vi "getLecServerList.vi"(8 "error in (no error)":errorcluster, 11 "SM1000-control in":T2) -> (0 "error out":errorcluster, 1 "Device identifiers":T1[](array[typedef]), 2 "piServerCount":i32, 3 "SM1000-control out":T2)   [LabVIEW 2013, in "SLMControl.lvlib" / "SM1000.lvclass"]
doc: "Get embedded controller device data.\n\nThis method returns a list of identifiers for the EC1000 modules for which valid broadcast packets have been received. One of the friendly names can be used in the method 'getBroadcastData' to obtain more extensive identification data.\nBecause of the asynchronous and periodic nature of the broadcast transmissions, it may take some time before all EC1000 controllers are recognized and reported via this method. Several successive calls may yield different results until enough time has passed to account for the longest broadcast interval. The broadcast interval is configured using the 'Session.requestFixedData' and 'Session.setFixedData' methods with the 'AdminConfig' data as an argument."
uses:
  SM1000.lvclass
  Object-reference.ctl
  Device-identification.ctl
  SM1000.lvclass/SM1000.ctl
  Custom-errors.ctl
  C:/Users/vangeste/Desktop/2015-06-02 - SLM - MAIF/HC-HardwareCharacterization/Sources/SM1000/LECBroadcast.dll
  HC-HardwareCharacterization/Sources/SM1000/LECBroadcast.dll
  DOTNET-error-int.vi
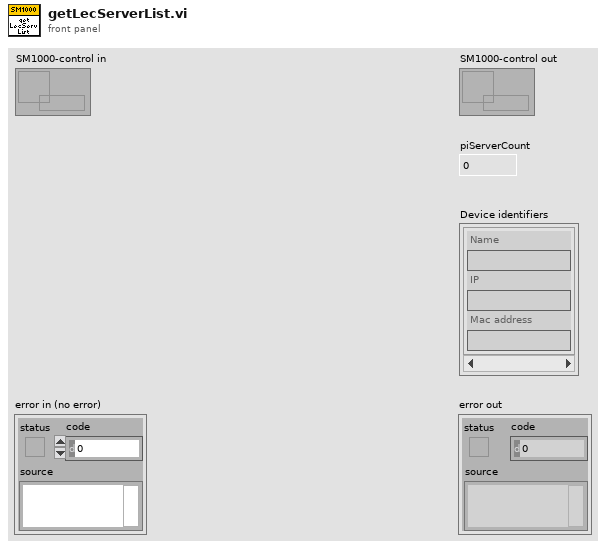
[diagram p1: front panel]
types:
  T1 = typedef "SLMControl.lvlib/SM1000.lvclass/Device-identification.ctl" = cluster{"Name":string, "IP":string, "Mac address":string}
  T2 = typedef "SLMControl.lvlib/SM1000.lvclass/Object-reference.ctl" = refnum<data-value>
  T3 = typedef "SLMControl.lvlib/SM1000.lvclass/Custom-errors.ctl" = enum16{"No error", "Not implemented", "Command not recognized", "Invalid input", "No connection", "Timeout", "Resource not loaded"}
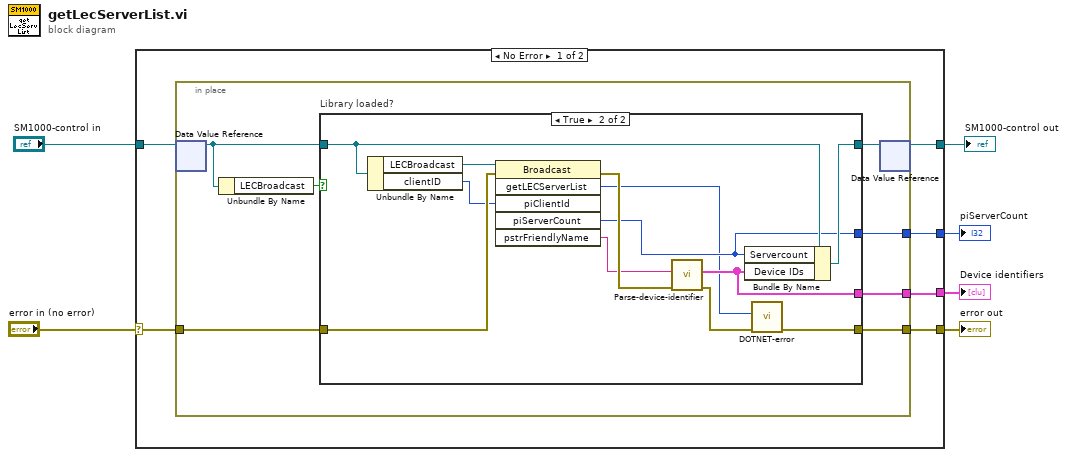
[diagram p0: block diagram]
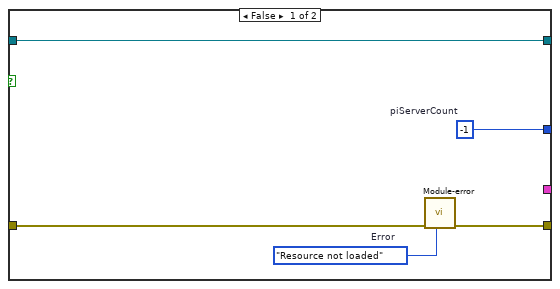
[diagram p2: hidden frame]
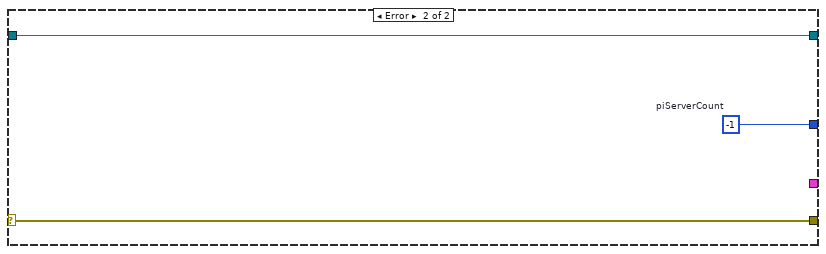
[diagram p3: hidden frame]
diagram:
  n1 = case shown="No Error" "error in (no error)" {
    selector: "error in (no error)" -> [w10 w39]
    tunnel: [w9 w39] -> w5
    tunnel: [w11 w38] -> w3
    tunnel: "SM1000-control in" -> [w12 w38]
    tunnel: [w8 _] -> w1
    tunnel: [w7 w37] -> w2
    frame No Error {
      n2 = in-place {
        in-place-border: w10 -> [w19]
        in-place-border: [w16] -> w9
        in-place-border: [w14] -> w8
        in-place-border: [w13] -> w7
        n3 = in-place-dvr #1(w12) -> (w17:refnum<class "SM1000.lvclass">)  [unwired: 1 out]
        n4 = Unbundle By Name(w17) -> ("LECBroadcast"=w18:bool)
        n5 = case "Library loaded?" shown="True" w18 {
          tunnel: w19 -> [w24 w34]
          tunnel: w17 -> [w22 w36]
          tunnel: [w23 w27] -> w16
          tunnel: [w22 w33] -> w15
          tunnel: [_ w29] -> w14
          tunnel: [w21 w28] -> w13
          frame False {
            w21 = -1  # piServerCount
            w20 = Custom-errors."Resource not loaded"  # Error
            n6 = call "Module-error.vi"("Error"=w20, "error in (no error)"=w24) -> ("error out"=w23:errorcluster)  [unwired: 9 in]
          }
          frame True {
            n7 = Unbundle By Name(w36) -> ("LECBroadcast"=w35:refnum<k24>, "clientID"=w32:i32)
            n8 = invoke class="Broadcast" method="getLECServerList"(reference=w35, error in=w34, "piClientId"=w32) -> (error out=w31:errorcluster, "getLECServerList"=w25:u32, "piServerCount"=w28:i32, "pstrFriendlyName"=w30:string)  [unwired: 3 in, 2 out]
            n9 = call "Parse-device-identifier.vi"("error in (no error)"=w31, "Multiple device identification XML string"=w30) -> ("error out"=w26:errorcluster, "Device identifiers"=w29:T1[])  [unwired: 8 in]
            n10 = Bundle By Name(cluster=w36, "Servercount"=w28, "Device IDs"=w29) -> (w33:refnum<class "SM1000.lvclass">)
            n11 = call-poly "DOTNET-error.vi"("error in (no error)"=w26, "Retun code"=w25) -> ("error out"=w27:errorcluster)  [unwired: 9 in]
          }
        }
        n12 = in-place-dvr #1(w15) -> (w11:T2)  [unwired: 1 out]
      }
    }
    frame Error {
      w37 = -1  # piServerCount
    }
  }
  "error out" <- w5
  "SM1000-control out" <- w3
  "piServerCount" <- w2
  "Device identifiers" <- w1
